vi "UpdateLotTable_New.vi"(8 "error in (no error)":errorcluster, 10 "input cluster":T1 {"50mA Data"."Current,mA" format="%_6g"; "50mA Data"."WL" format="%_6g"; "50mA Data"."Voltage" format="%_6g"; "50mA Data"."Power" format="%_6g"; "20mA Data"."Reverse" format="%#_3g"; "20mA Data"."Current,mA" format="%_6g"; "20mA Data"."Knee Current" format="%#_3g"; "20mA Data"."WL" format="%_6g"; "20mA Data"."Voltage" format="%_6g"; "20mA Data"."Power" format="%_5g"}, 11 "LotData in":refnum<class "LotData.lvclass">) -> (0 "error out":errorcluster, 3 "LotData out":refnum<class "LotData.lvclass">)   [LabVIEW 2012, in "LotData.lvclass"]
uses:
  LotData.lvclass
  Controls/TestData.ctl
  LotData.lvclass/LotData.ctl
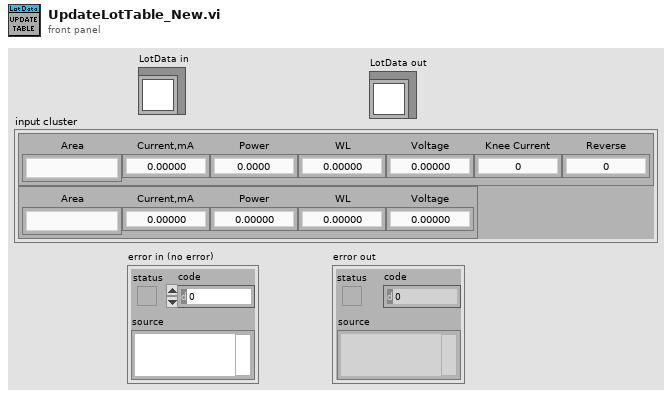
[diagram p1: front panel]
types:
  T1 = typedef "TestData.ctl" = cluster{"20mA Data":cluster{"Area":string, "Current,mA":dbl, "Power":dbl, "WL":dbl, "Voltage":dbl, "Knee Current":dbl, "Reverse":dbl}, "50mA Data":cluster{"Area":string, "Current,mA":dbl, "Power":dbl, "WL":dbl, "Voltage":dbl}}
  T2 = cluster{"Area":string, "Current,mA":dbl, "Power":dbl, "WL":dbl, "Voltage":dbl, "Knee Current":dbl, "Reverse":dbl}
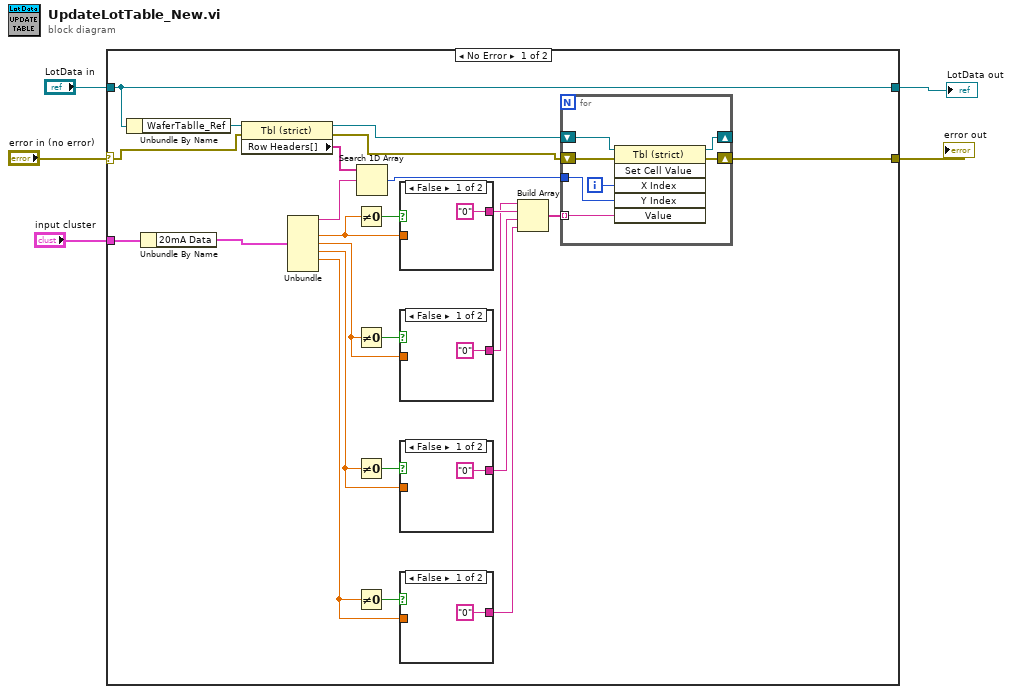
[diagram p0: block diagram]
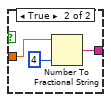
[diagram p2: hidden frame]
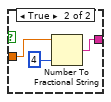
[diagram p3: hidden frame]
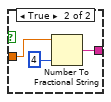
[diagram p4: hidden frame]
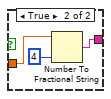
[diagram p5: hidden frame]
diagram:
  n1 = case shown="No Error" "error in (no error)" {
    selector: "error in (no error)" -> [w7 w54]
    tunnel: [w28 w54] -> w4
    tunnel: [w27 w53] -> w2
    tunnel: "LotData in" -> [w27 w53]
    tunnel: "input cluster" -> [w8 _]
    frame No Error {
      n2 = Unbundle By Name(w27) -> ("WaferTablle_Ref"=w29:refnum<vi>)
      n3 = Unbundle By Name(w8) -> ("20mA Data"=w26:T2)
      n4 = property class="Tbl (strict)"(reference=w29, error in=w7) -> (reference out=w23:refnum<vi>, error out=w6:errorcluster, "Row Headers[]"=w25:string[])
      n5 = Unbundle(w26) -> ("Area"=w24:string, "Power"=w19:dbl, "WL"=w13:dbl, "Voltage"=w14:dbl, "Knee Current"=w15:dbl)  [unwired: 2 out]
      n6 = Not Equal To 0?(x=w19) -> (x != 0?=w20:bool)
      n7 = Not Equal To 0?(x=w13) -> (x != 0?=w18:bool)
      n8 = Not Equal To 0?(x=w14) -> (x != 0?=w17:bool)
      n9 = Not Equal To 0?(x=w15) -> (x != 0?=w16:bool)
      n10 = Search 1D Array(1D array=w25, element=w24) -> (index of element=w22:i32)  [unwired: 1 in]
      n11 = case shown="False" w20 {
        tunnel: w19 -> [_ w45]
        tunnel: ["0" ("F-format string") w43] -> w12
        frame False {
        }
        frame True {
          n12 = Number To Fractional String(number=w45, precision (6)=i16 4) -> (F-format string=w43:string)  [unwired: 2 in]
        }
      }
      n13 = case shown="False" w18 {
        tunnel: ["0" ("F-format string") w40] -> w11
        tunnel: w13 -> [_ w39]
        frame False {
        }
        frame True {
          n14 = Number To Fractional String(number=w39, precision (6)=i16 4) -> (F-format string=w40:string)  [unwired: 2 in]
        }
      }
      n15 = case shown="False" w17 {
        tunnel: ["0" ("F-format string") w36] -> w10
        tunnel: w14 -> [_ w35]
        frame False {
        }
        frame True {
          n16 = Number To Fractional String(number=w35, precision (6)=i16 4) -> (F-format string=w36:string)  [unwired: 2 in]
        }
      }
      n17 = case shown="False" w16 {
        tunnel: ["0" ("F-format string") w32] -> w9
        tunnel: w15 -> [_ w31]
        frame False {
        }
        frame True {
          n18 = Number To Fractional String(number=w31, precision (6)=i16 4) -> (F-format string=w32:string)  [unwired: 2 in]
        }
      }
      n19 = Build Array(w11, w12, w10, w9) -> (w21:string[])
      n20 = for {
        tunnel: w21 -> [w49] mode=indexing
        tunnel: w22 -> [w51]
        shift-right: [w47] -> w28
        shift-left: w6 -> [w48]
        shift-right: [w46] -> _
        shift-left: w23 -> [w52]
        i -> [w50]
        n21 = invoke class="Tbl (strict)" method="Set Cell Value"(reference=w52, error in=w48, "X Index"=w50, "Y Index"=w51, "Value"=w49) -> (reference out=w46:refnum<vi>, error out=w47:errorcluster)  [unwired: 1 in, 4 out]
      }
    }
    frame Error {
    }
  }
  "error out" <- w4
  "LotData out" <- w2
